vi "Constructor Basic.vi"(6 "Controller Config":refnum<class "Panel Form Controller Configuration.lvclass">, 8 "error in (no error)":errorcluster, 9 "Panel Logic":refnum<class "Model Panel Logic.lvclass">, 10 "Panel Form Controller":refnum<class "Panel Form Controller.lvclass">, 11 "Form Model Configuration in":refnum<class "Form Model Configuration.lvclass">) -> (0 "error out":errorcluster, 3 "Form Model Configuration out":refnum<class "Form Model Configuration.lvclass">)   [LabVIEW 2020, in "Form Model.lvlib" / "Form Model Configuration.lvclass"]
uses:
  Form Model Configuration.lvclass
  Forms Controller/Form Controller/Panel Form Controller.lvclass
  Forms Controller/Configuration/Controller Configuration/Panel Form Controller Configuration.lvclass
  Form Model Interfaces/Model Panel Logic Interface/Model Panel Logic.lvclass
  Forms Controller/Configuration/Controller Configuration/Panel Form Controller Configuration.lvclass/Panel Form Controller Configuration.ctl
  Forms Controller/Form Controller/Panel Form Controller.lvclass/Panel Form Controller.ctl
  Form Model Configuration.lvclass/Form Model Configuration.ctl
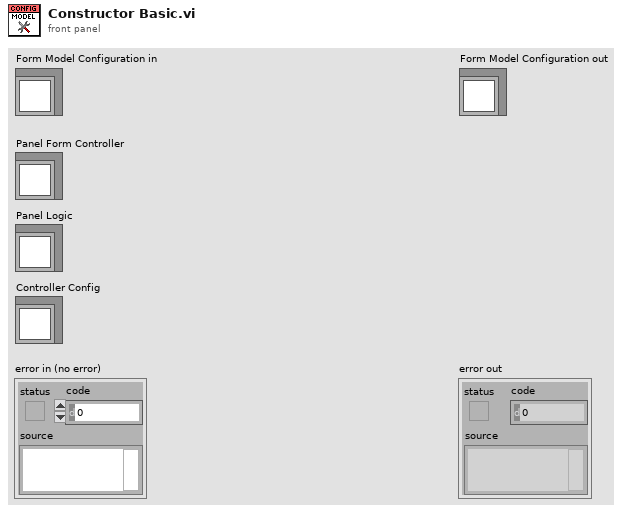
[diagram p1: front panel]
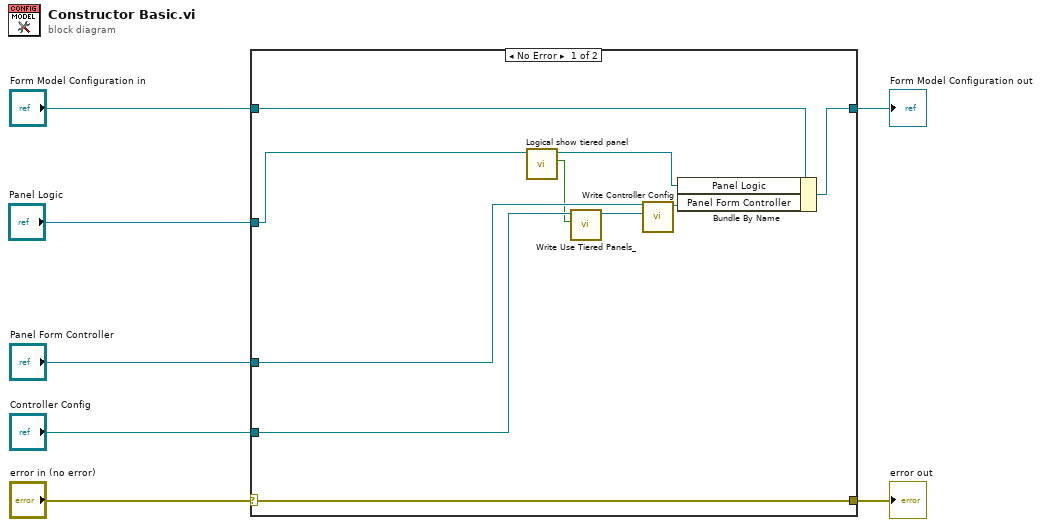
[diagram p0: block diagram]
diagram:
  n1 = case shown="No Error" "error in (no error)" {
    selector: "error in (no error)" -> [w17 w19]
    tunnel: [w17 w19] -> w6
    tunnel: [w16 w18] -> w4
    tunnel: "Form Model Configuration in" -> [w15 w18]
    tunnel: "Panel Form Controller" -> [w14 _]
    tunnel: "Controller Config" -> [w12 _]
    tunnel: "Panel Logic" -> [w9 _]
    frame No Error {
      n2 = call-dynamic "Logical show tiered panel.vi"("Model Panel Logic in"=w9) -> ("Show tiered panel?"=w10:bool, "Model Panel Logic out"=w8:refnum<class "Model Panel Logic.lvclass">)  [unwired: 8 in, 1 out]
      n3 = call "Write Use Tiered Panels_.vi"("Use Tiered Panels?"=w10, "Panel Form Controller Configuration in"=w12) -> ("Panel Form Controller Configuration out"=w11:refnum<class "Panel Form Controller Configuration.lvclass">)  [unwired: 8 in, 1 out]
      n4 = call "Write Controller Config.vi"("Controller Config"=w11, "Panel Form Controller in"=w14) -> ("Panel Form Controller out"=w13:refnum<class "Panel Form Controller.lvclass">)  [unwired: 8 in, 1 out]
      n5 = Bundle By Name(cluster=w15, "Panel Logic"=w8, "Panel Form Controller"=w13) -> (w16:refnum<class "Form Model Configuration.lvclass">)
    }
    frame Error {
    }
  }
  "error out" <- w6
  "Form Model Configuration out" <- w4
